vi "Configure Line Feed.vi"(8 "error in (no error)":errorcluster, 11 "Tovey9150 in":refnum<class "Tovey 9150.lvclass">) -> (0 "error out":errorcluster, 3 "Tovey9150 out":refnum<class "Tovey 9150.lvclass">)   [LabVIEW 2015, in "Tovey 9150.lvclass"]
uses:
  Tovey 9150.lvclass
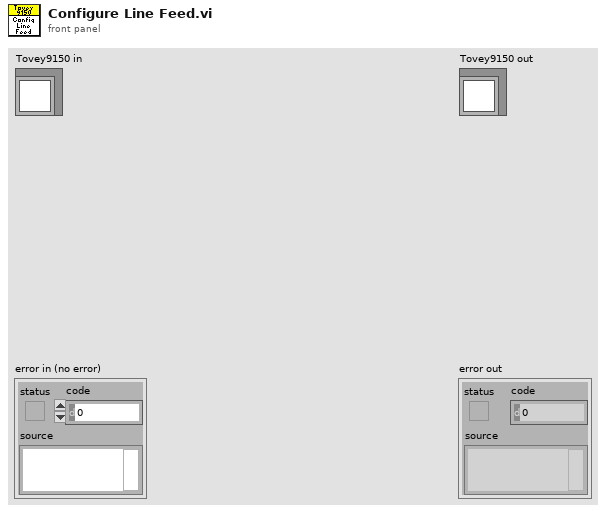
[diagram p1: front panel]
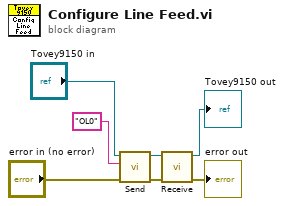
[diagram p0: block diagram]
diagram:
  n1 = call "Send.vi"("error in (no error)"="error in (no error)", "Message"="OL0", "Tovey9150 in"="Tovey9150 in") -> ("error out"=w3:errorcluster, "Tovey9150 out"=w4:refnum<class "Tovey 9150.lvclass">)  [unwired: 7 in]
  n2 = call "Receive.vi"("error in (no error)"=w3, "Tovey9150 in"=w4) -> ("error out"=→"error out":errorcluster, "Tovey9150 out"=→"Tovey9150 out":refnum<class "Tovey 9150.lvclass">)  [unwired: 7 in, 1 out]
